vi "Set Recipients2.vi"(0 "handles cluster in":T1 caption="ハンドルクラスター入力", 5 "to":string[](array[string]) caption="受信者", 7 "cc":string[](array[string]), 9 "bcc":string[](array[string]), 11 "error in (no error)":errorcluster caption="エラー入力（エラーなし）") -> (4 "handles cluster out":T1 caption="ハンドルクラスター出力", 15 "error out":errorcluster caption="エラー出力")   [LabVIEW 2015]
doc: "Eメールを受け取る受信者リストを設定します。"
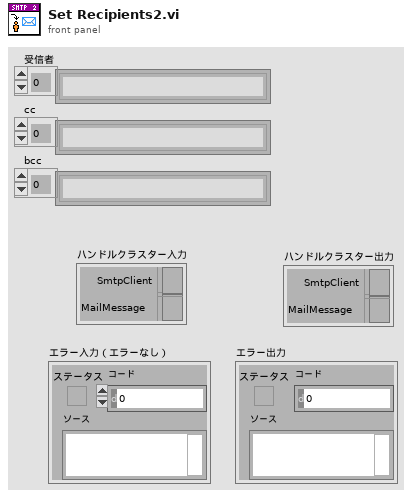
[diagram p1: front panel]
types:
  T1 = cluster{"SmtpClient":refnum<k24>, "MailMessage":refnum<k24>}
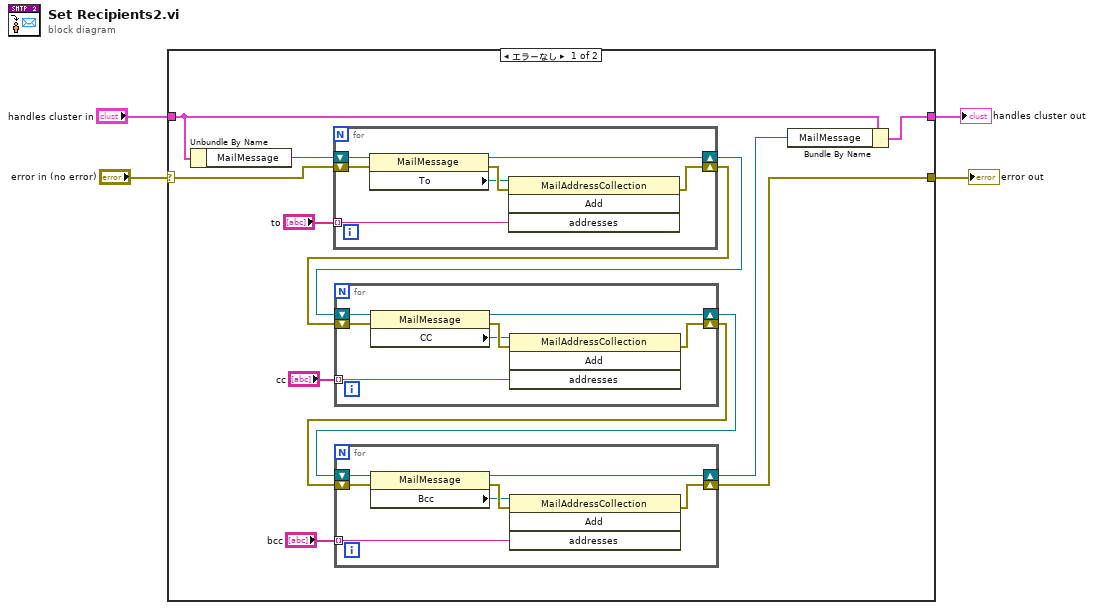
[diagram p0: block diagram]
diagram:
  n1 = case shown="エラーなし" "error in (no error)" {
    selector: "error in (no error)" -> [w15 w40]
    tunnel: [w6 w40] -> w3
    tunnel: "handles cluster in" -> [w8 w39]
    tunnel: [w5 w39] -> w1
    frame No Error {
      n2 = Unbundle By Name(w8) -> ("MailMessage"=w16:refnum<k24>)
      n3 = for {
        tunnel: "to" -> [w35] mode=indexing
        shift-right: [w33] -> w14
        shift-left: w15 -> [w34]
        shift-right: [w32] -> w13
        shift-left: w16 -> [w38]
        n4 = property class="MailMessage"(reference=w38, error in=w34) -> (reference out=w32:refnum<k24>, error out=w37:errorcluster, "To"=w36:refnum<k24>)
        n5 = invoke class="MailAddressCollection" method="Add"(reference=w36, error in=w37, "addresses"=w35) -> (error out=w33:errorcluster)  [unwired: 1 in, 3 out]
      }
      n6 = for {
        tunnel: "cc" -> [w28] mode=indexing
        shift-right: [w26] -> w11
        shift-left: w14 -> [w27]
        shift-right: [w25] -> w10
        shift-left: w13 -> [w31]
        n7 = property class="MailMessage"(reference=w31, error in=w27) -> (reference out=w25:refnum<k24>, error out=w30:errorcluster, "CC"=w29:refnum<k24>)
        n8 = invoke class="MailAddressCollection" method="Add"(reference=w29, error in=w30, "addresses"=w28) -> (error out=w26:errorcluster)  [unwired: 1 in, 3 out]
      }
      n9 = for {
        tunnel: "bcc" -> [w21] mode=indexing
        shift-right: [w19] -> w6
        shift-left: w11 -> [w20]
        shift-right: [w18] -> w7
        shift-left: w10 -> [w24]
        n10 = property class="MailMessage"(reference=w24, error in=w20) -> (reference out=w18:refnum<k24>, error out=w23:errorcluster, "Bcc"=w22:refnum<k24>)
        n11 = invoke class="MailAddressCollection" method="Add"(reference=w22, error in=w23, "addresses"=w21) -> (error out=w19:errorcluster)  [unwired: 1 in, 3 out]
      }
      n12 = Bundle By Name(cluster=w8, "MailMessage"=w7) -> (w5:T1)
    }
    frame Error {
    }
  }
  "handles cluster out" <- w1
  "error out" <- w3
